vi "Unpack Control Drag Ended.vi"(0 "ControlDragEndedMsg In":refnum<class "ControlDragEndedMsg.lvclass">) -> (4 "Ctl Refnum":refnum<vi>, 6 "Control Label":string, 8 "Time":u32, 10 "Result":enum16{"Drop Cancel", "Drop Move", "Drop Copy"}(ring))   [LabVIEW 2017, in "ActorEvents.lvlib" / "ControlDragEndedMsg.lvclass"]
doc: "<License>\nCopyright © 2017 Composed Systems, LLC | All rights reserved\nwww.composed.io\n\nAuthor: Ethan Stern <ethan.stern@composed.io>\n\nThis software is provided \"AS IS\" WITHOUT WARRANTIES, either express or implied, AND IS FOR EDUCATIONAL PURPOSES ONLY.\n</License>"
uses:
  ControlDragEndedMsg.lvclass
  ControlDragEndedMsg.lvclass/ControlDragEndedMsg.ctl
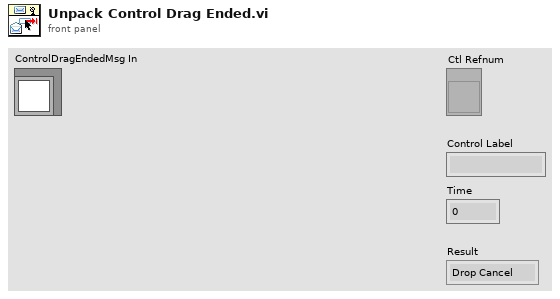
[diagram p1: front panel]
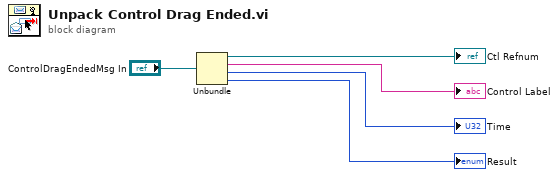
[diagram p0: block diagram]
diagram:
  n1 = Unbundle("ControlDragEndedMsg In") -> (→"Ctl Refnum":refnum<vi>, →"Control Label":string, →"Time":u32, →"Result":enum16{"Drop Cancel", "Drop Move", "Drop Copy"})
